vi "Ref Counter.vi"(0 "Ref Count in":u32, 1 "Ref Counter Action Enum":T1) -> (2 "Ref Count out":u32)   [LabVIEW 2021]
uses:
  <vilib>/myRIO/Common/Instrument Driver Framework/Utilities/typedefs/Ref Counter Action Enum.ctl
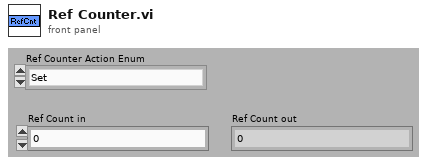
[diagram p1: front panel]
types:
  T1 = typedef "Ref Counter Action Enum.ctl" = enum16{"Set", "Get", "Increment", "Decrement"}
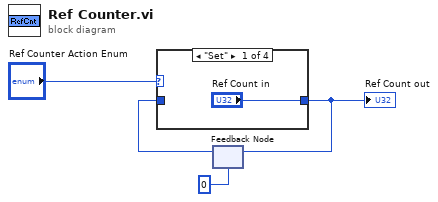
[diagram p0: block diagram]
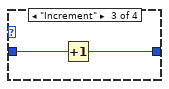
[diagram p3: hidden frame]
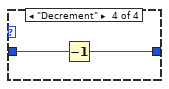
[diagram p4: hidden frame]
diagram:
  n1 = feedback #1(u32 0 ("RefCount in")) -> (w3:u32)
  n2 = case shown="\"Set\"" "Ref Counter Action Enum" {
    tunnel: ["Ref Count in" w6 w7 w10] -> w4
    tunnel: w3 -> [_ w6 w8 w9]
    frame "Set" {
    }
    frame "Get" {
    }
    frame "Increment" {
      n3 = Increment(x=w8) -> (x+1=w7:u32)
    }
    frame "Decrement" {
      n4 = Decrement(x=w9) -> (x-1=w10:u32)
    }
  }
  "Ref Count out" <- w4
  n5 = feedback-in #1(w4) -> ()
